vi "FPGA_VoltageDividingIndicator.vi"() -> ()   [LabVIEW 2014]
uses:
  <vilib>/rvi/Emulation/niFpgaGetClockAttributes.vi
  <vilib>/rvi/Emulation/niFpgaSctlEmulationGetInTimedLoop.vi
  <vilib>/rvi/Emulation/niFpgaEmulationReportErrorSimple.vi
  <vilib>/rvi/eio/common/nirviEmuTemplateMethod_errors.vi
  <vilib>/rvi/Emulation/niFpgaCriticalErrorInLSC.vi
  <vilib>/eio/EIONode/EIONode.xnode
panel:
  in  "stop":bool
  in  "AO2":i16
  in  "AO1":i16
  in  "AO0":i16
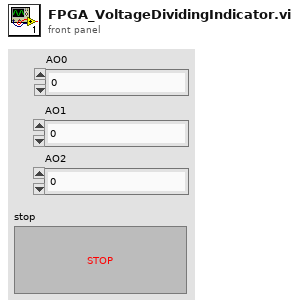
[diagram p1: front panel]
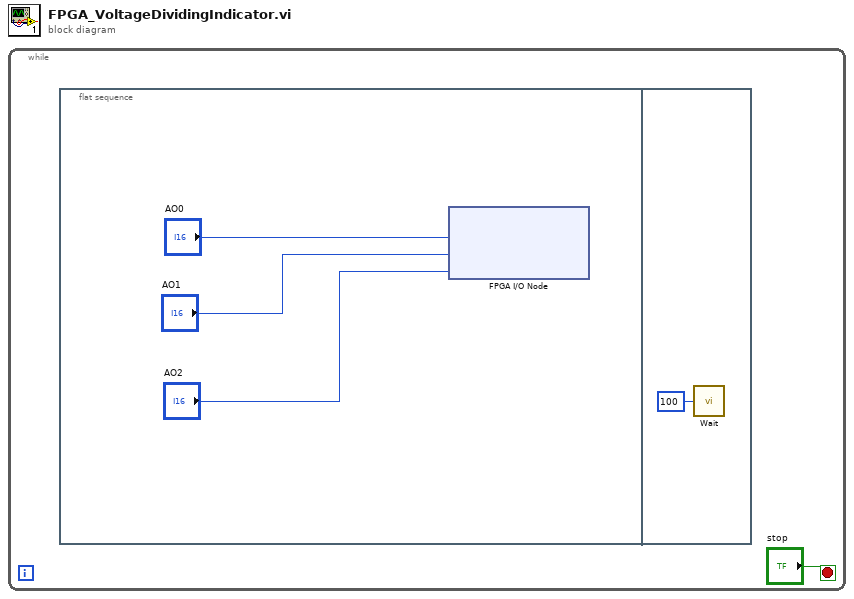
[diagram p0: block diagram]
diagram:
  n1 = while {
    stop <- "stop" stop-if-true
    n2 = flat-sequence {
      frame #0 {
        n3 = xnode "FPGA I/O Node"("Connector0/AO0"="AO0", "Connector0/AO1"="AO1", "Connector0/AO2"="AO2") -> ()  [unwired: 3 in, 3 out]
      }
      frame #1 {
        n4 = call "Wait"("Count(uSec)"=u32 100) -> ()  [unwired: 1 out]
      }
    }
  }
